vi "Segment Log File (Time).vi"(8 "error in (no error)":errorcluster, 11 "Time Segmented Log in":refnum<class "Time Segmented Log.lvclass">) -> (0 "error out":errorcluster, 2 "Segment Log File":bool, 3 "Time Segmented Log out":refnum<class "Time Segmented Log.lvclass">)   [LabVIEW 2012, in "Waveform Data Logger Engine.lvlib" / "Time Segmented Log.lvclass"]
uses:
  Time Segmented Log.lvclass
  Segmented Log/Segmented Log.lvclass/Segmented Log.ctl
  Log Files/Log File/Log File.lvclass/Log File.ctl
  Time Segmented Log.lvclass/Time Segmented Log.ctl
  Segmented Log/Segmented Log.lvclass
  Log Files/Log File/Log File.lvclass
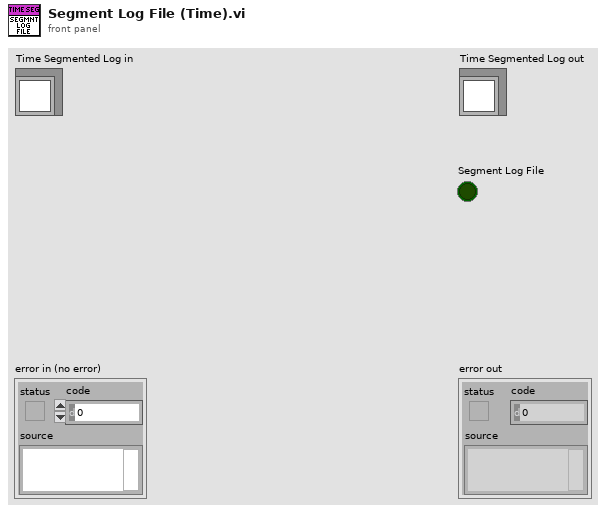
[diagram p1: front panel]
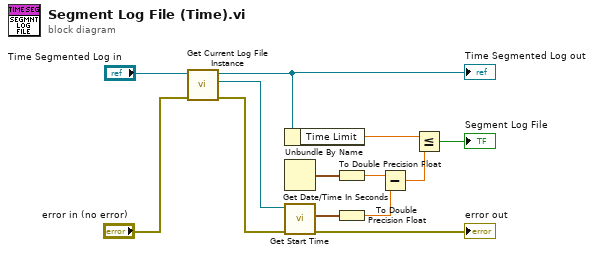
[diagram p0: block diagram]
diagram:
  n1 = call "Get Current Log File Instance.vi"("error in (no error)"="error in (no error)", "Segmented Log in"="Time Segmented Log in") -> ("error out"=w7:errorcluster, "Log File Instance"=w8:refnum<class "Log File.lvclass">, "Segmented Log out"=w9:refnum<class "Time Segmented Log.lvclass">)  [unwired: 7 in]
  "Time Segmented Log out" <- w9
  n2 = Unbundle By Name(w9) -> ("Time Limit"=w11:dbl)
  n3 = Get Date/Time In Seconds() -> (seconds since 1Jan1904=w13:timestamp)
  n4 = call "Get Start Time.vi"("error in (no error)"=w7, "Log File in"=w8) -> ("error out"=→"error out":errorcluster, "Start Time"=w6:timestamp)  [unwired: 7 in, 1 out]
  n5 = To Double Precision Float(number=w13) -> (double precision float=w2:dbl)
  n6 = To Double Precision Float(number=w6) -> (double precision float=w1:dbl)
  n7 = Subtract(x=w2, y=w1) -> (x-y=w12:dbl)
  n8 = Less Or Equal?(x=w11, y=w12) -> (x <= y?=→"Segment Log File":bool)
